vi "EminemDashRead.vi"   [LabVIEW 2023]
uses:
  <vilib>/Rock Robotics/Network Tables/NT Read Number.vi
  EminemGlobals.vi
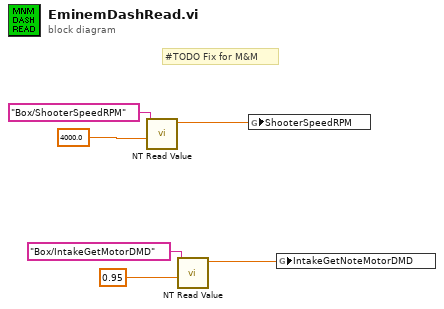
[diagram p0: block diagram]
diagram:
  # "#TODO Fix for M&M"
  n1 = call-poly <vilib>:"NT Read Value.vi"("default value"=4000.0, "name"="Box/ShooterSpeedRPM") -> ("value"=w2:dbl)  [unwired: 7 in, 2 out]
  n2 = call-poly <vilib>:"NT Read Value.vi"("default value"=0.95, "name"="Box/IntakeGetMotorDMD") -> ("value"=w1:dbl)  [unwired: 7 in, 2 out]
  n3 = global write "EminemGlobals.vi" "ShooterSpeedRPM"(w2) -> ()
  n4 = global write "EminemGlobals.vi" "IntakeGetNoteMotorDMD"(w1) -> ()
